vi "Configure Modulation (Frequency).vi"(4 "Peak Deviation (100.00 Hz)":dbl=100.0, 6 "Modulation Frequency (100.00 Hz)":dbl=100.0, 7 "Enable Frequency Modulation (T:Enable)":bool=TRUE, 8 "error in (no error)":errorcluster, 9 "Modulation Waveform (0: Sine)":u16(ring) items=["Sine", "Square", "Triangle"], 10 "FM Source (0: Internal)":u16(ring) items=["Internal", "External"], 11 "VISA resource name":refnum<visa-resource-name>) -> (0 "error out":errorcluster, 3 "VISA resource name out":refnum<visa-resource-name>)   [LabVIEW 2013, in "Template - Function Generator.lvlib"]
doc: "Configures and enables frequency modulation (FM). In FM, the frequency of the carrier is varied by the frequency of the modulating waveform. \n\n<B>Note:</B> The carrier waveform shape and parameters are set by the Configure Standard Waveform VI."
uses:
  <instrlib>/_Template - Function Generator/Template - Function Generator.lvlib
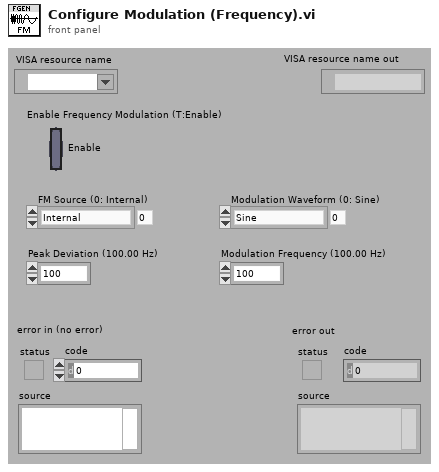
[diagram p1: front panel]
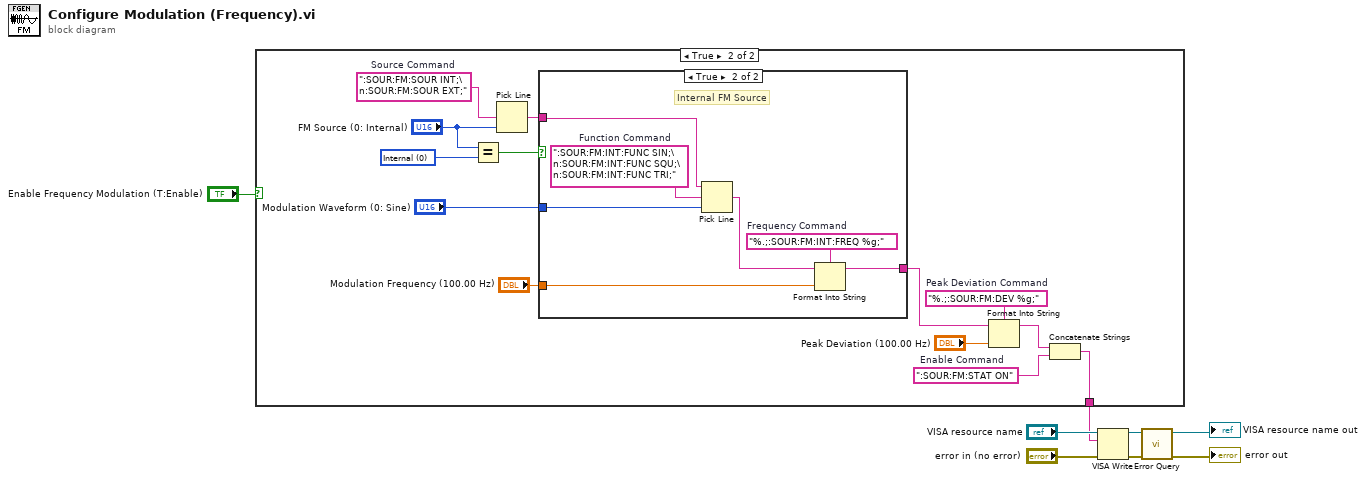
[diagram p0: block diagram]
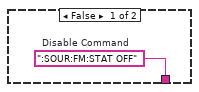
[diagram p2: hidden frame]
diagram:
  n1 = case shown="True" "Enable Frequency Modulation (T:Enable)" {
    tunnel: [w9 w12] -> w6
    frame False {
      w9 = ":SOUR:FM:STAT OFF"  # Disable Command
    }
    frame True {
      w10 = ":SOUR:FM:STAT ON"  # Enable Command
      w18 = u16 0 items=["Internal", "External"] ("Source (0: Internal)")
      w17 = ":SOUR:FM:SOUR INT;\n:SOUR:FM:SOUR EXT;"  # Source Command
      w21 = "%.;:SOUR:FM:DEV %g;"  # Peak Deviation Command
      n2 = Equal?(x="FM Source (0: Internal)", y=w18) -> (x = y?=w15:bool)
      n3 = Pick Line(multi-line string=w17, line index="FM Source (0: Internal)") -> (output string=w14:string)  [unwired: 1 in]
      n4 = case shown="True" w15 {
        tunnel: [w23 w28] -> w20
        tunnel: "Modulation Frequency (100.00 Hz)" -> [_ w27]
        tunnel: w14 -> [w23 w25]
        tunnel: "Modulation Waveform (0: Sine)" -> [_ w24]
        frame False {
          # "External FM Source"
          # "EDIT: If external modulation is configurable,\ncall the external modulation command."
        }
        frame True {
          w26 = ":SOUR:FM:INT:FUNC SIN;\n:SOUR:FM:INT:FUNC SQU;\n:SOUR:FM:INT:FUNC TRI;"  # Function Command
          w30 = "%.;:SOUR:FM:INT:FREQ %g;"  # Frequency Command
          # "Internal FM Source"
          n5 = Pick Line(string ("")=w25, multi-line string=w26, line index=w24) -> (output string=w29:string)
          n6 = Format Into String(format string=w30, initial string=w29, w27) -> (resulting string=w28:string)  [unwired: 1 in, 1 out]
        }
      }
      n7 = Format Into String(format string=w21, initial string=w20, "Peak Deviation (100.00 Hz)") -> (resulting string=w11:string)  [unwired: 1 in, 1 out]
      n8 = Concatenate Strings(w11, w10) -> (w12:string)
    }
  }
  n9 = VISA Write(VISA resource name="VISA resource name", write buffer=w6, error in (no error)="error in (no error)") -> (VISA resource name out=w4:refnum<visa-resource-name>, error out=w5:errorcluster)  [unwired: 1 out]
  n10 = call <instrlib>:"Error Query.vi"("error in (no error)"=w5, "VISA resource name"=w4) -> ("error out"=→"error out":errorcluster, "VISA resource name out"=→"VISA resource name out":refnum<visa-resource-name>)  [unwired: 6 in, 2 out]
